vi "Determine Possible Moves.vi"(8 "error in (no error)":errorcluster, 11 "Reversi in":refnum<class "Reversi.lvclass">) -> (0 "error out":errorcluster, 3 "Reversi out":refnum<class "Reversi.lvclass">)   [LabVIEW 2020, in "Reversi.lvlib" / "Reversi.lvclass"]
uses:
  Reversi.lvclass
  Turn Enum.ctl
  Space Ring.ctl
  Reversi.lvclass/Reversi.ctl
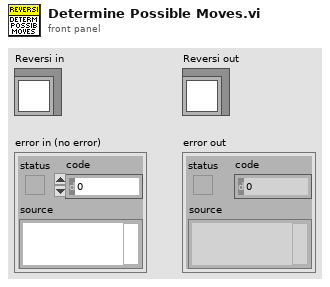
[diagram p1: front panel]
types:
  T1 = typedef "Reversi.lvlib/Reversi.lvclass/Space Ring.ctl" = u16
  T2 = typedef "Reversi.lvlib/Reversi.lvclass/Turn Enum.ctl" = enum16{"Black", "White"}
  T3 = typedef "Reversi.lvlib/Reversi.lvclass/Space Coordinates.ctl" = cluster{"Row":i32, "Column":i32}
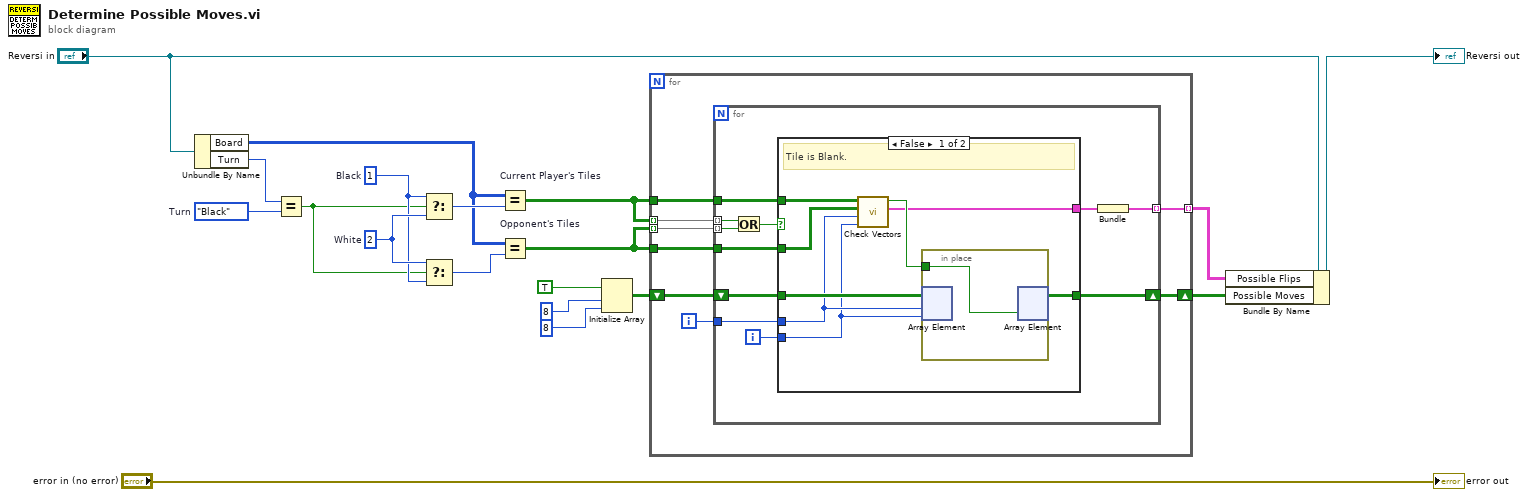
[diagram p0: block diagram]
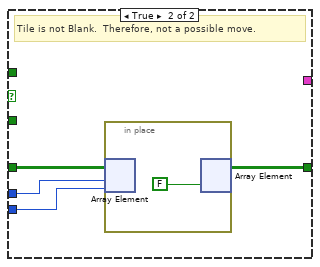
[diagram p2: hidden frame]
diagram:
  w11 = T1 2  # White
  w10 = T1 1  # Black
  w7 = Turn_Enum."Black"  # Turn
  n1 = Unbundle By Name("Reversi in") -> ("Board"=w3:T1[][], "Turn"=w2:T2)
  n2 = Equal?(x=w2, y=w7) -> (x = y?=w8:bool)
  n3 = Select(t=w10, s=w8, f=w11) -> (s? t:f=w17:T1)
  n4 = Select(t=w11, s=w8, f=w10) -> (s? t:f=w9:T1)
  n5 = Equal? "Current Player's Tiles"(x=w3, y=w17) -> (x = y?=w6:bool[][])
  n6 = Equal? "Opponent's Tiles"(x=w3, y=w9) -> (x = y?=w5:bool[][])
  n7 = Initialize Array(TRUE, 8, 8) -> (w13:bool[][])
  n8 = for {
    tunnel: w6 -> [w26]
    tunnel: w5 -> [w25]
    shift-right: [w23] -> w12
    shift-left: w13 -> [w24]
    tunnel: w6 -> [w22] mode=indexing
    tunnel: w5 -> [w21] mode=indexing
    tunnel: [w20] -> w4 mode=indexing
    i -> [w27]
    n9 = for {
      tunnel: w27 -> [w37]
      tunnel: w26 -> [w33]
      tunnel: w25 -> [w34]
      shift-right: [w35] -> w23
      shift-left: w24 -> [w36]
      tunnel: w22 -> [w32] mode=indexing
      tunnel: w21 -> [w31] mode=indexing
      tunnel: [w28] -> w20 mode=indexing
      i -> [w38]
      n10 = Or(x=w32, y=w31) -> (x .or. y?=w30:bool)
      n11 = case shown="False" w30 {
        tunnel: w38 -> [w41 w49]
        tunnel: w37 -> [w42 w50]
        tunnel: w36 -> [w46 w51]
        tunnel: [w45 w48] -> w35
        tunnel: w34 -> [w43 _]
        tunnel: w33 -> [w44 _]
        tunnel: [w39 _] -> w29
        frame False {
          # "Tile is Blank."
          n12 = call "Check Vectors.vi"("Column"=w41, "Row"=w42, "Opponent's Tiles"=w43, "Current Player's Tiles"=w44) -> ("Possible Flips"=w39:cluster{T3[]}[], "Possible Location"=w40:bool)  [unwired: 6 in]
          n13 = in-place {
            in-place-border: w40 -> [w47]
            n14 = in-place-array #1(w46, w42, w41) -> ()  [unwired: 1 out]
            n15 = in-place-array #1(w47) -> (w45:bool[][])  [unwired: 2 out]
          }
        }
        frame True {
          # "Tile is not Blank.  Therefore, not a possible move."
          n16 = in-place {
            n17 = in-place-array #2(w51, w50, w49) -> ()  [unwired: 1 out]
            n18 = in-place-array #2(FALSE) -> (w48:bool[][])  [unwired: 2 out]
          }
        }
      }
      n19 = Bundle("Possible Flips"=w29) -> (w28:cluster{"Possible Flips":cluster{T3[]}[]})  [unwired: 1 in]
    }
  }
  n20 = Bundle By Name(cluster="Reversi in", "Possible Flips"=w4, "Possible Moves"=w12) -> (→"Reversi out":refnum<class "Reversi.lvclass">)
  "error out" <- "error in (no error)"
